vi "test Parse DBL Array3.vi"(11 "Test Case In":refnum<class "Test Named Fields Parser.lvclass">) -> (0 "error out":errorcluster, 3 "Test Case Out":refnum<class "Test Named Fields Parser.lvclass">)   [LabVIEW 2024, in "Test Named Fields Parser.lvclass"]
uses:
  Test Named Fields Parser.lvclass
  C:/Program Files/National Instruments/LabVIEW 2025/vi.lib/Astemes/LUnit/Test Case.lvclass
  CSV Parser/Named Fields Parser/Named Fields Parser.lvclass
  <vilib>/Astemes/LUnit/Test Case.lvclass/Test Case.ctl
  <vilib>/Astemes/LUnit/Append Fail Result.vi
  <vilib>/Astemes/LUnit/Append Pass Result.vi
  <vilib>/Astemes/LUnit/Run In UI.vi
  <vilib>/Astemes/LUnit/Test Case.lvclass
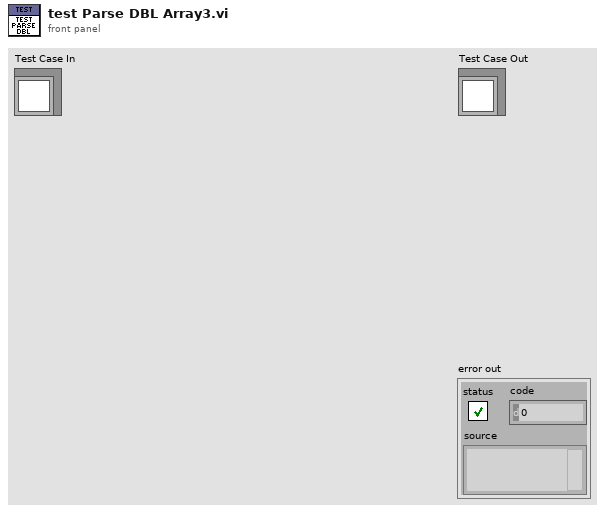
[diagram p1: front panel]
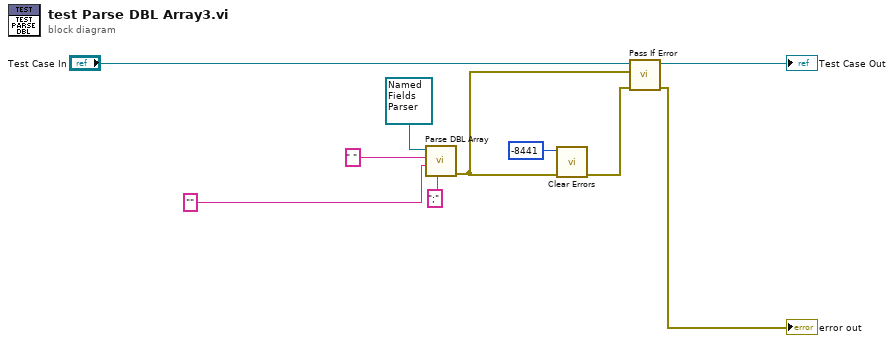
[diagram p0: block diagram]
diagram:
  n1 = call-dynamic "Parse DBL Array.vi"("Seperator"=";", "Input <JSON>"="", "csv string"=" ", "Named Columns Parser in"=refnum<class "Named Fields Parser.lvclass"> refnum) -> ("error out"=w4:errorcluster)  [unwired: 5 in, 2 out]
  n2 = call <vilib>:"Clear Errors.vi"("error in (no error)"=w4, "specific error code to clear (0: all)"=-8441) -> ("error out"=w3:errorcluster)  [unwired: 4 in, 1 out]
  n3 = call <vilib>:"Pass If Error.vi"("error in (no error)"=w3, "Assert error"=w4, "LUnit Test Case In"="Test Case In") -> ("error out"=→"error out":errorcluster, "LUnit Test Case Out"=→"Test Case Out":refnum<class "Test Named Fields Parser.lvclass">)  [unwired: 7 in]
